vi "fanPIP.vi"(8 "error in (no error)":errorcluster) -> (0 "error out":errorcluster, 3 "FAN-18":string)   [LabVIEW 2018]
uses:
  Global_usbComm.vi
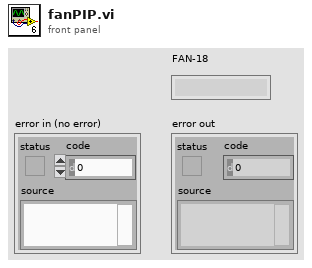
[diagram p1: front panel]
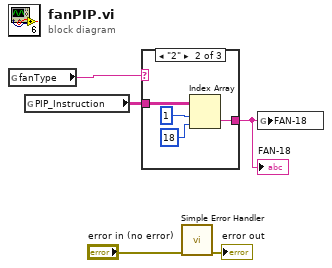
[diagram p0: block diagram]
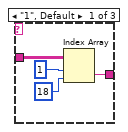
[diagram p2: hidden frame]
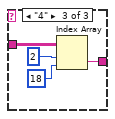
[diagram p3: hidden frame]
diagram:
  n1 = global read "Global_usbComm.vi" "fanType"() -> (w1:string)
  n2 = global read "Global_usbComm.vi" "PIP_Instruction"() -> (w2:string[][])
  n3 = case shown="\"2\"" w1 {
    tunnel: w2 -> [w7 w11 w16]
    tunnel: [w6 w10 w14] -> w3
    frame "1", Default {
      n4 = Index Array(array=w7, index (row)=1 ("disabled index (row)"), index (col)=18 ("disabled index (col)")) -> (element=w6:string)
    }
    frame "2" {
      n5 = Index Array(array=w11, index (row)=1 ("disabled index (row)"), index (col)=18 ("disabled index (col)")) -> (element=w10:string)
    }
    frame "4" {
      n6 = Index Array(array=w16, index (row)=2 ("disabled index (row)"), index (col)=18 ("disabled index (col)")) -> (element=w14:string)
    }
  }
  "FAN-18" <- w3
  n7 = call <vilib>:"Simple Error Handler.vi"("error in (no error)"="error in (no error)") -> ("error out"=→"error out":errorcluster)  [unwired: 4 in, 4 out]
  n8 = global write "Global_usbComm.vi" "FAN-18"(w3) -> ()
